vi "Read_binary_data.vi"() -> (1 "PWA Binary":i16[][](array[numeric]), 3 "PWA Frequency Hz":dbl format="%.2f", 5 "EOF?":bool, 6 "Block Header":string)   [LabVIEW 2022 SP3]
uses:
  Controls/Read I16 data cluster.ctl
  Globals/Meas_global.vi
  Globals/LDA_global.vi
panel:
  out "svnBaseRevision":u32
  out "string":string
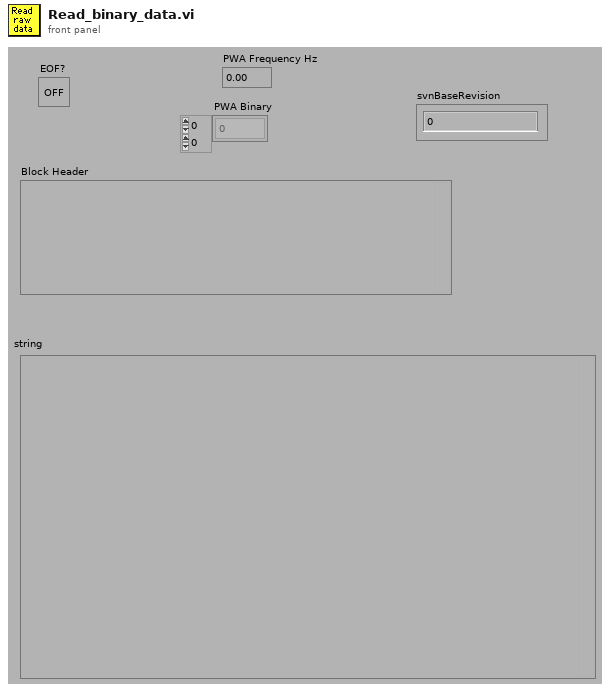
[diagram p1: front panel]
types:
  T1 = typedef "Analysis_info_cluster.ctl" = cluster{"Colour":u32, "Inst type":T2, "Inst name":string, "Symbol":string, "Code name":string, "Extra Info":string, "Inst Array":T3, "U":dbl, "u^2":dbl, "u^3":dbl, "u^4":dbl, "Skew_u":dbl, "Kurt_u":dbl, "Sd Error in Mean":dbl, "% u'/U":dbl, "X":dbl, "Y":dbl, "Z":dbl, "Timescale integral Estimate":dbl, "Sd Error in Variance":dbl, "Calib File":path, "Calib Constants":dbl[], "Output Position":bool, "Stats":enum16{"None", "Basic", "Full"}, "Av Sampling Rate":dbl, "Av No of Samples":dbl, "Total Meas Time (s)":dbl, "OrigChName":string, "Max value":dbl, "Min value":dbl, "Req Sample Rate Hz":dbl, "Sync Delay Time (s)":dbl, "Ch No":i16, "Device":string, "Use Latest Calib":bool, "Port":string, "Metadata Ch Names":string[], "Metadata Ch Values":string[], "Label":string, "chState":T4, "Point Drift":dbl, "inputConfig":string}
  T2 = typedef "Inst_type.ctl" = enum16{"Raw voltage", "Raw with zero offsetting", "Propeller anemometer", "Pressure Transducer", "Pitot-static tube", "Hot wire", "Cross wire 1", "Cross wire 2", "Generic Linear", "Generic Polynomial", "Generic BackPoly", "Fast FID", "Thermocouple", "Cold wire", "Pulsed Wire", "LDA Vel", "LDA Tran time", "LDA Arr time", "Microphone"}
  T3 = typedef "Instrument_Array.ctl" = enum16{"PWA", "LDA", "Analogue"}
  T4 = typedef "channelState.ctl" = enum32{"No Selection", "Solo", "Mute"}
  T5 = enum16{"read/write", "read-only", "write-only", "write-only (truncate)"}
  T6 = typedef "Read I16 data cluster.ctl" = cluster{"scale multiplier":dbl, "scale offset":dbl, "Length":i32, "Sampling rate (Hz)":dbl, "Sync Delay (s)":dbl}
  T7 = typedef "BSA_Type.ctl" = enum16{"57N11", "BSA F60"}
  T8 = typedef "PWA_Data.ctl" = enum16{"No PWA Data", "One Ch PWA"}
  T9 = typedef "Time_Trace_Cluster.ctl" = cluster{"Weighting":dbl[], "Voltage":dbl[], "Eng Values":dbl[]}
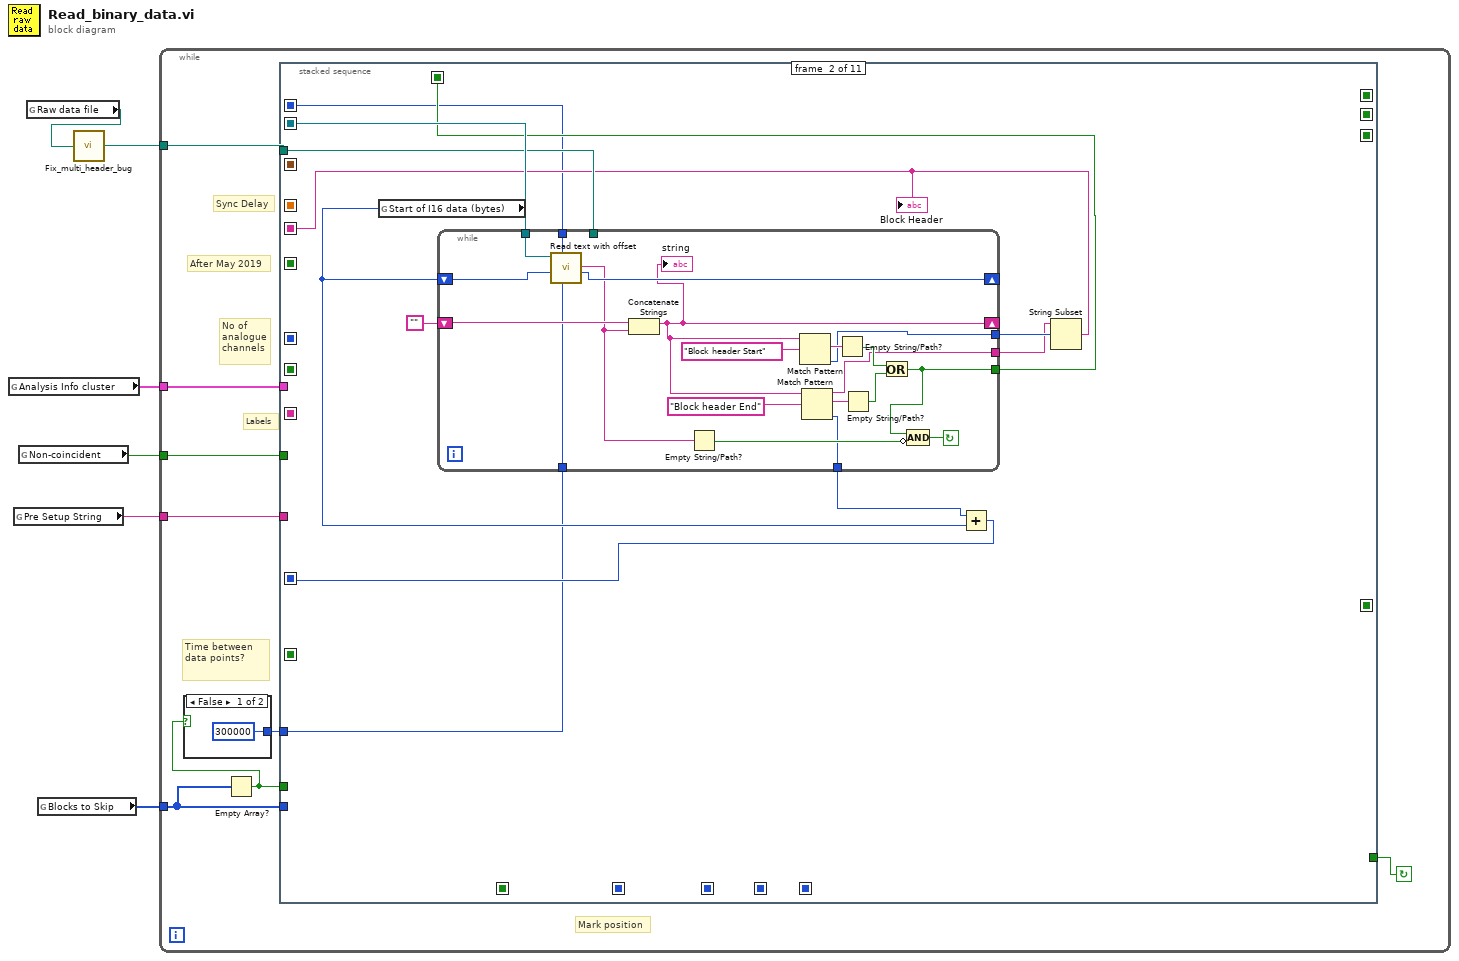
[diagram p0: block diagram]
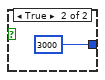
[diagram p2: hidden frame]
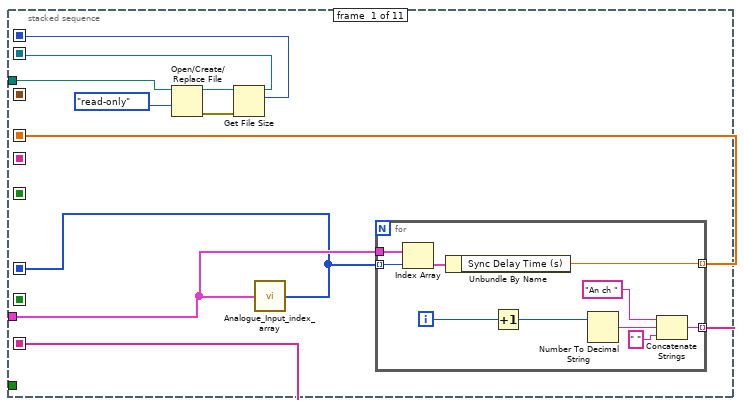
[diagram p3: hidden frame]
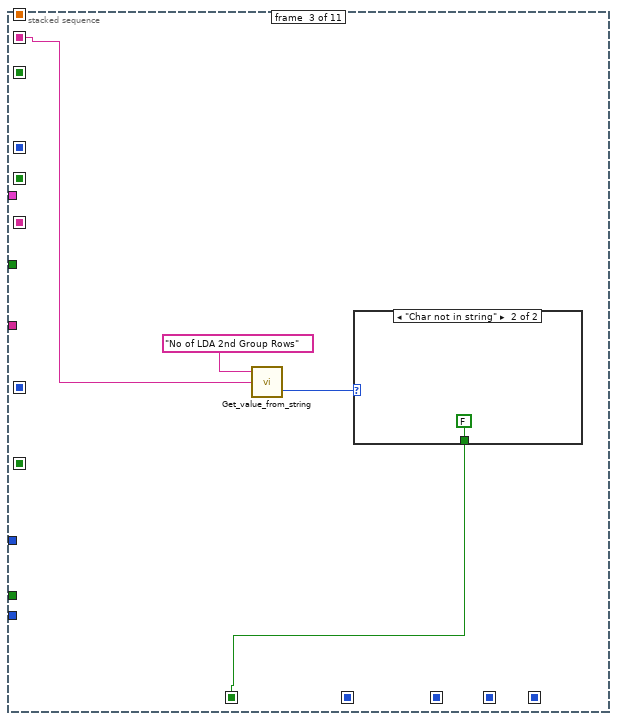
[diagram p4: hidden frame]
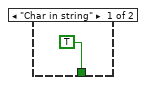
[diagram p5: hidden frame]
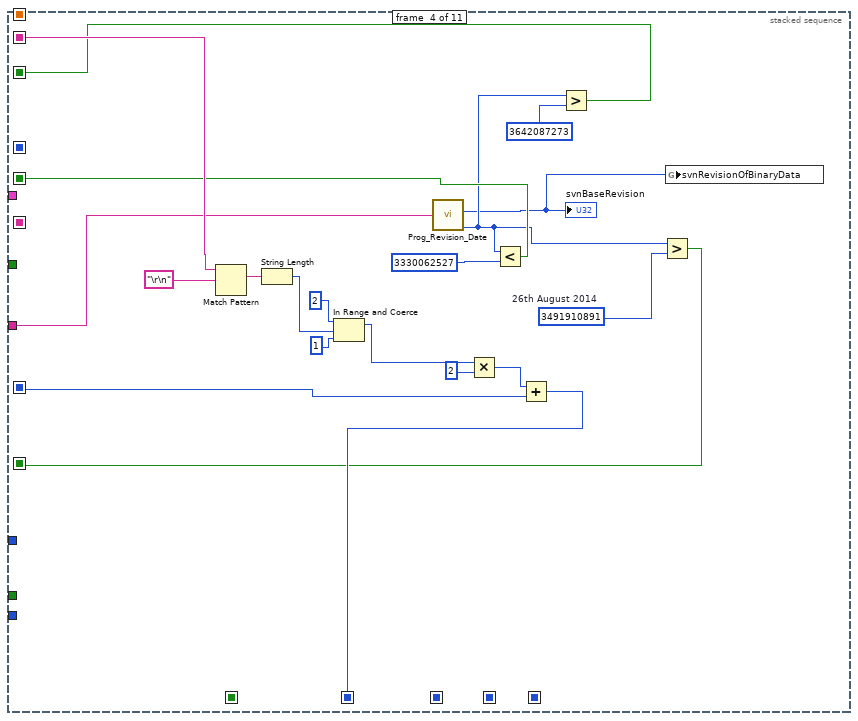
[diagram p6: hidden frame]
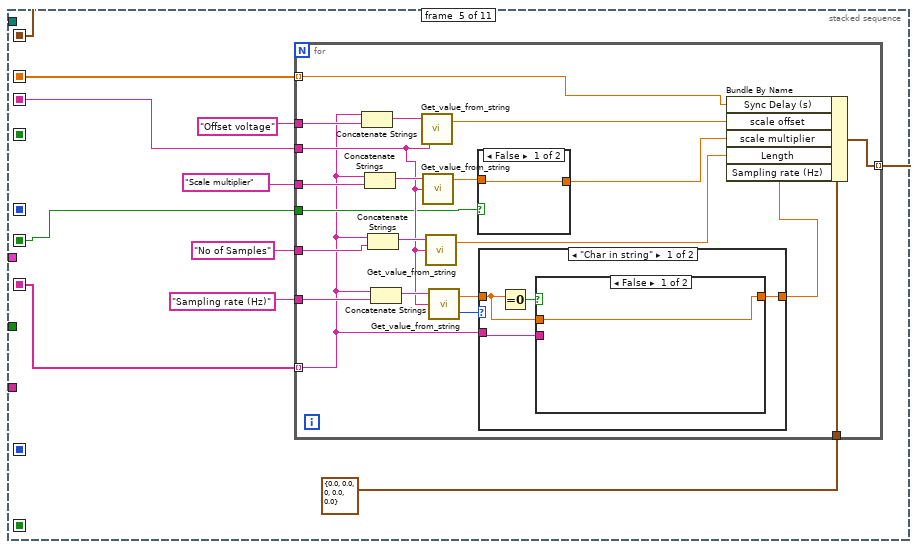
[diagram p7: hidden frame]
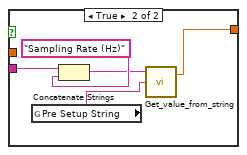
[diagram p8: hidden frame]
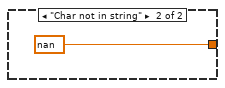
[diagram p9: hidden frame]
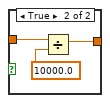
[diagram p10: hidden frame]
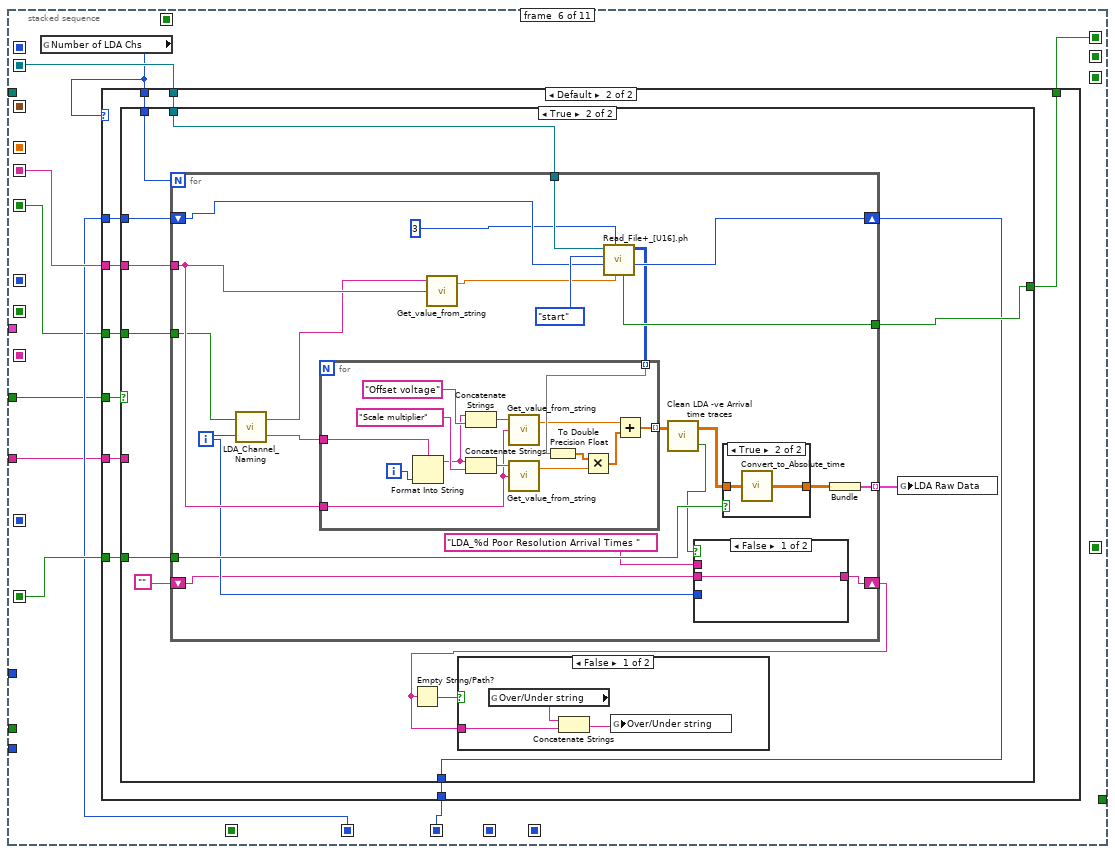
[diagram p11: hidden frame]
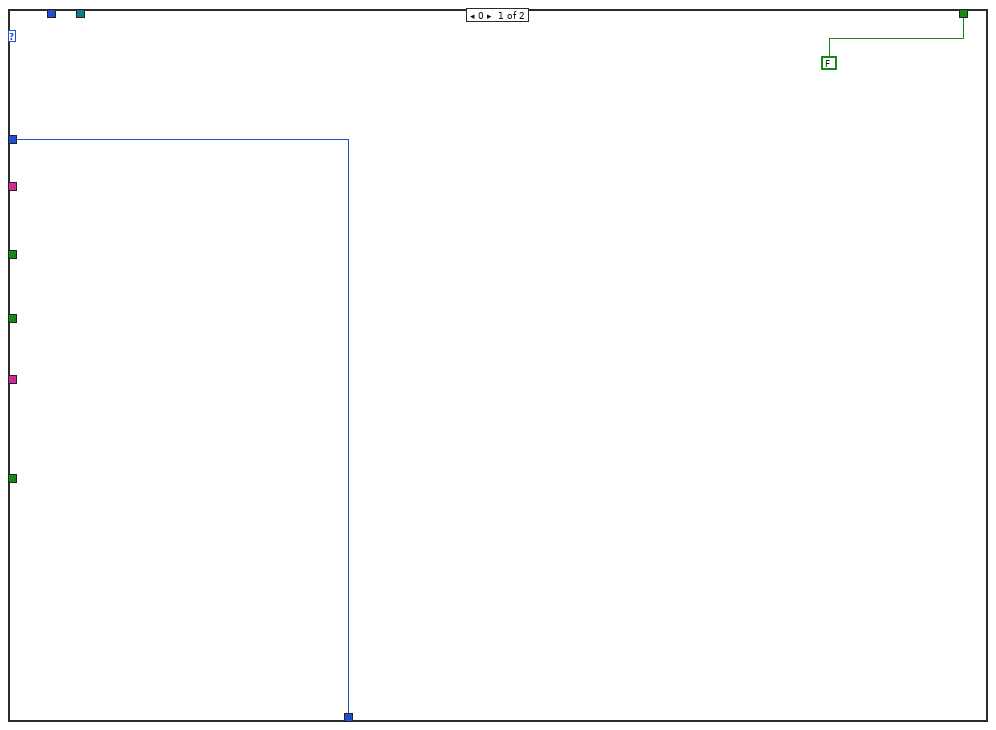
[diagram p12: hidden frame]
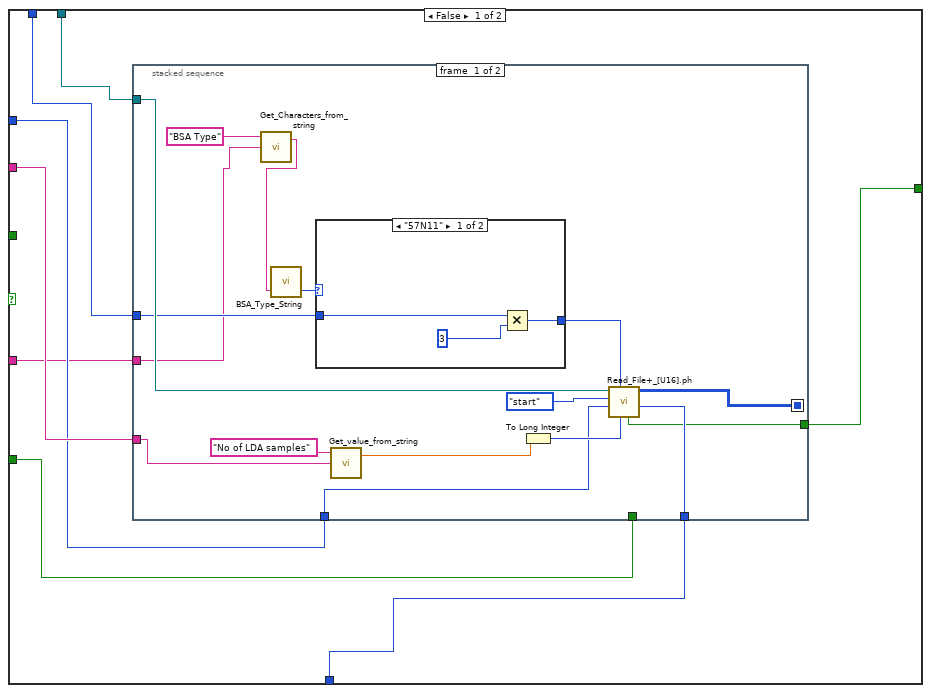
[diagram p13: hidden frame]
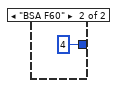
[diagram p14: hidden frame]
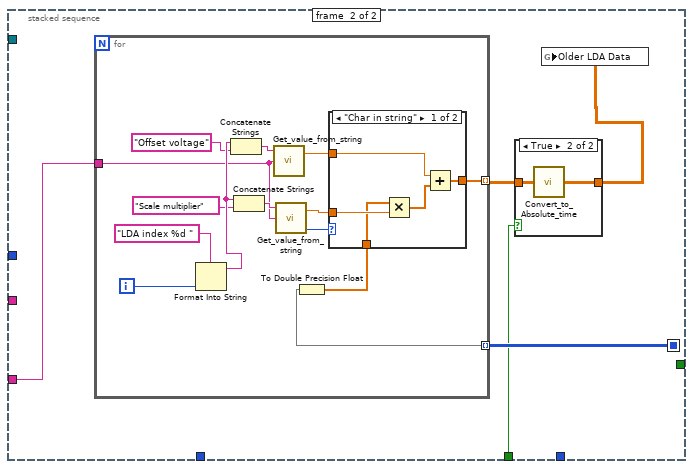
[diagram p15: hidden frame]
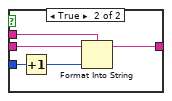
[diagram p19: hidden frame]
diagram:
  n1 = global read "Meas_global.vi" "Analysis Info cluster"() -> (w4:T1[])
  n2 = global read "Meas_global.vi" "Pre Setup String"() -> (w2:string)
  n3 = global read "LDA_global.vi" "Non-coincident"() -> (w3:bool)
  n4 = global read "Meas_global.vi" "Raw data file"() -> (w6:path)
  n5 = global read "Meas_global.vi" "Blocks to Skip"() -> (w1:i32[])
  n6 = call "Fix_multi_header_bug.vi"("Raw data File to Read"=w6) -> ("Raw data File to Read Out"=w5:path)
  n7 = while {
    tunnel: w5 -> [w14]
    tunnel: w4 -> [w12]
    tunnel: w3 -> [w11]
    tunnel: w2 -> [w10]
    tunnel: w1 -> [w9]
    stop <- w13 continue-if-true
    # "After May 2019"
    # "Sync Delay"
    # "Time between data points?"
    # "Mark position"
    # "Labels"
    # "No of\nanalogue\nchannels"
    n8 = Empty Array?(array=w9) -> (empty?=w8:bool)
    n9 = case shown="False" w8 {
      tunnel: [300000 3000] -> w7
      frame False {
      }
      frame True {
      }
    }
    n10 = stacked-sequence {
      seq-local: [w19 _ _ _ _ _ _ _ _ _ _] -> [_ w48 _ _ _ w148 w286 w325 _ w361 w416]
      seq-local: [_ w39 _ _ _ _ _ _ _ _ _] -> [_ _ w71 w88 w100 w149 w288 w320 w341 _ _]
      seq-local: [w21 _ _ _ _ _ _ _ _ _ _] -> [_ _ _ _ _ _ _ w319 _ _ _]
      seq-local: [w24 _ _ _ _ _ _ _ _ _ _] -> [_ _ _ _ w102 _ _ _ _ _ _]
      seq-local: [_ _ _ w92 _ _ _ _ _ _ _] -> [_ _ _ _ _ w147 _ _ _ _ _]
      seq-local: [_ _ _ _ _ w145 _ _ _ _ _] -> [_ _ _ _ _ _ w281 _ _ _ _]
      seq-local: [_ _ _ _ _ _ w287 _ _ _ _] -> [_ _ _ _ _ _ _ w323 _ _ _]
      seq-local: [_ w44 _ _ _ _ _ _ _ _ _] -> [_ _ _ _ _ _ _ _ _ _ w417]
      seq-local: [_ w43 _ _ _ _ _ _ _ _ _] -> [_ _ _ w93 _ _ _ _ _ _ _]
      seq-local: [_ _ _ _ _ _ _ _ w340 _ _] -> [_ _ _ _ _ _ _ _ _ w354 _]
      seq-local: [_ _ _ _ _ _ _ w322 _ _ _] -> [_ _ _ _ _ _ _ _ _ w358 _]
      seq-local: [_ _ w69 _ _ _ _ _ _ _ _] -> [_ _ _ _ _ _ _ _ _ _ _]
      seq-local: [_ _ _ w81 _ _ _ _ _ _ _] -> [_ _ _ _ _ w150 _ _ _ _ _]
      seq-local: [_ _ _ w80 _ _ _ _ _ _ _] -> [_ _ _ _ w99 _ _ _ _ _ _]
      seq-local: [_ _ _ _ w96 _ _ _ _ _ _] -> [_ _ _ _ _ _ _ w316 _ _ _]
      seq-local: [w23 _ _ _ _ _ _ _ _ _ _] -> [_ _ _ _ w95 _ _ _ _ _ _]
      seq-local: [_ _ _ w77 _ _ _ _ _ _ _] -> [_ _ _ _ _ w146 _ _ _ _ _]
      seq-local: [w17 _ _ _ _ _ _ _ _ _ _] -> [_ w38 _ _ _ _ _ _ _ w359 _]
      seq-local: [_ _ _ _ _ w141 _ _ _ _ _] -> [_ _ _ _ _ _ w279 _ _ _ _]
      seq-local: [_ _ _ _ _ _ w280 _ _ _ _] -> [_ _ _ _ _ _ _ w314 _ _ _]
      seq-local: [_ _ _ _ _ _ _ w315 _ _ _] -> [_ _ _ _ _ _ _ _ _ w356 _]
      tunnel: w14 -> [w25 w47 _ _ _ _ _ _ _ w360 w418]
      tunnel: [_ _ _ _ _ _ _ _ _ w353 _] -> w13
      tunnel: w12 -> [w22 _ _ _ _ _ _ _ _ _ _]
      tunnel: w11 -> [_ _ _ _ _ w144 _ _ _ _ _]
      tunnel: w10 -> [_ _ _ w76 _ w143 _ _ _ _ _]
      tunnel: w9 -> [_ _ _ _ _ _ _ _ w339 w352 _]
      tunnel: w8 -> [_ _ _ _ _ _ _ _ w338 w351 _]
      tunnel: w7 -> [_ w37 _ _ _ _ _ _ _ w350 _]
      frame #0 {
        n11 = Open/Create/Replace File(file path (use dialog)=w25, access (0:read/write)=T5."read-only" ("open mode (0)")) -> (refnum out=w20:refnum<file>, error out=w18:errorcluster)  [unwired: 1 in, 4 out]
        n12 = Get File Size(file=w20, error in=w18) -> (refnum out=w19:refnum<file>, size (in bytes)=w17:i64)  [unwired: 1 out]
        n13 = call "Analogue_Input_index_array.vi"("Analysis Info cluster"=w22) -> ("Array"=w21:i32[])
        n14 = for {
          tunnel: [w35] -> w24 mode=indexing
          tunnel: [w34] -> w23 mode=indexing
          tunnel: w22 -> [w29]
          tunnel: w21 -> [w28] mode=indexing
          i -> [w36]
          n15 = Index Array(array=w29, index=w28) -> (element=w27:T1)
          n16 = Unbundle By Name(w27) -> ("Sync Delay Time (s)"=w34:dbl)
          n17 = Increment(x=w36) -> (x+1=w31:i32)
          n18 = Number To Decimal String(number=w31) -> (decimal integer string=w33:string)  [unwired: 1 out]
          n19 = Concatenate Strings("An ch ", w33, " ") -> (w35:string)
        }
      }
      frame #1 {
        n20 = global read "Meas_global.vi" "Start of I16 data (bytes)"() -> (w45:i64)
        n21 = while {
          tunnel: [w55] -> w42
          tunnel: [w56] -> w44
          shift-left: "" -> [w59]
          shift-right: [w52] -> _
          tunnel: w47 -> [_]
          tunnel: w48 -> [w66]
          shift-left: w45 -> [w62]
          shift-right: [w65] -> _
          tunnel: [w54] -> w40
          tunnel: [w51] -> w41
          tunnel: w38 -> [w50]
          tunnel: w37 -> [w49]
          stop <- w63 continue-if-true
          n22 = call "Read text with offset.vi"("Count"=w49, "File Size"=w50, "Start of read offset (chars.: 0)"=w62, "Refnum In"=w66) -> ("Mark after Read"=w65:i64, "text"=w53:string)  [unwired: 3 in, 3 out]
          n23 = Concatenate Strings(w59, w53) -> (w52:string)
          "string" <- w52
          n24 = Empty String/Path?(string/path=w53) -> (empty?=w64:bool)
          n25 = Match Pattern(string=w52, regular expression="Block header Start") -> (match substring=w61:string, offset past match=w51:i32)  [unwired: 3 out]
          n26 = Match Pattern(string=w52, regular expression="Block header End") -> (before substring=w54:string, match substring=w67:string, offset past match=w55:i32)  [unwired: 2 out]
          n27 = Empty String/Path?(string/path=w61) -> (empty?=w58:bool)
          n28 = Empty String/Path?(string/path=w67) -> (empty?=w57:bool)
          n29 = Or(x=w58, y=w57) -> (x .or. y?=w56:bool)
          n30 = Compound Arithmetic op=AND(w56, invert w64) -> (w63:bool)
        }
        n31 = Add(x=w42, y=w45) -> (x+y=w43:i64)
        n32 = String Subset(string=w40, offset (0)=w41) -> (substring=w39:string)  [unwired: 1 out]
        "Block Header" <- w39
      }
      frame #2 {
        n33 = call "Get_value_from_string.vi"("Input string"=w71, "Variable name"="No of LDA 2nd Group Rows") -> ("Status"=w70:enum16{"Char in string", "Char not in string"})  [unwired: 1 in, 1 out]
        n34 = case shown="\"Char not in string\"" w70 {
          tunnel: [TRUE FALSE] -> w69
          frame "Char in string" {
          }
          frame "Char not in string" {
          }
        }
      }
      frame #3 {
        w82 = u32 3491910891  # 26th August 2014
        n35 = Match Pattern(string=w88, regular expression="\r\n") -> (match substring=w87:string)  [unwired: 4 out]
        n36 = String Length(string=w87) -> (length=w86:i32)
        n37 = In Range and Coerce(upper limit=2, x=w86, lower limit=1) -> (coerced(x)=w85:i32)  [unwired: 1 out]
        n38 = call "Prog_Revision_Date.vi"("Input string"=w76) -> ("Revision time (s)"=w79:u32, "svnBaseRevision"=w75:u32)  [unwired: 3 out]
        "svnBaseRevision" <- w75
        n39 = Multiply(x=w85, y=2) -> (x*y=w91:i32)
        n40 = Less?(x=w79, y=u32 3330062527 ("unsigned 32bit integer")) -> (x < y?=w80:bool)
        n41 = Add(x=w91, y=w93) -> (x+y=w92:i64)
        n42 = Greater?(x=w79, y=u32 3642087273 ("unsigned 32bit integer")) -> (0:w77:bool)
        n43 = Greater?(x=w79, y=w82) -> (0:w81:bool)
        n44 = global write "Meas_global.vi" "svnRevisionOfBinaryData"(w75) -> ()
      }
      frame #4 {
        n45 = for {
          tunnel: "Scale multiplier" -> [w125]
          tunnel: "Offset voltage" -> [w124]
          tunnel: w100 -> [w116]
          tunnel: w102 -> [w106] mode=indexing
          tunnel: T6 {"scale multiplier"=0.0, "scale offset"=0.0, "Length"=0, "Sampling rate (Hz)"=0.0, "Sync Delay (s)"=0.0} -> [w121]
          tunnel: "Sampling rate (Hz)" ("string") -> [w118]
          tunnel: "No of Samples" -> [w117]
          tunnel: w99 -> [w115]
          tunnel: [w108] -> w96 mode=indexing
          tunnel: w95 -> [w107] mode=indexing
          n46 = Concatenate Strings(w106, w124) -> (w123:string)
          n47 = Concatenate Strings(w106, w125) -> (w122:string)
          n48 = Concatenate Strings(w106, w117) -> (w120:string)
          n49 = Concatenate Strings(w106, w118) -> (w119:string)
          n50 = call "Get_value_from_string.vi"("Input string"=w116, "Variable name"=w123) -> ("Value"=w113:dbl)  [unwired: 1 in, 1 out]
          n51 = call "Get_value_from_string.vi"("Input string"=w116, "Variable name"=w122) -> ("Value"=w114:dbl)  [unwired: 1 in, 1 out]
          n52 = call "Get_value_from_string.vi"("Input string"=w116, "Variable name"=w120) -> ("Value"=w111:dbl)  [unwired: 1 in, 1 out]
          n53 = call "Get_value_from_string.vi"("Input string"=w116, "Variable name"=w119) -> ("Status"=w110:enum16{"Char in string", "Char not in string"}, "Value"=w109:dbl)  [unwired: 1 in]
          n54 = case shown="False" w115 {
            tunnel: w114 -> [w137 w140]
            tunnel: [w137 w138] -> w112
            frame False {
            }
            frame True {
              n55 = Divide(x=w140, y=10000.0) -> (x/y=w138:dbl)
            }
          }
          n56 = case shown="\"Char in string\"" w110 {
            tunnel: [w127 nan ("Value")] -> w105
            tunnel: w109 -> [w126 _]
            tunnel: w106 -> [w129 _]
            frame "Char in string" {
              n57 = Equal To 0?(x=w126) -> (x = 0?=w128:bool)
              n58 = case shown="False" w128 {
                tunnel: w129 -> [_ w135]
                tunnel: [w130 w131] -> w127
                tunnel: w126 -> [w130 _]
                frame False {
                }
                frame True {
                  n59 = global read "Meas_global.vi" "Pre Setup String"() -> (w133:string)
                  n60 = Concatenate Strings(w135, "Sampling Rate (Hz)" ("string")) -> (w132:string)
                  n61 = call "Get_value_from_string.vi"("Input string"=w133, "Variable name"=w132) -> ("Value"=w131:dbl)  [unwired: 1 in, 1 out]
                }
              }
            }
            frame "Char not in string" {
            }
          }
          n62 = Bundle By Name(cluster=w121, "Sync Delay (s)"=w107, "scale offset"=w113, "scale multiplier"=w112, "Length"=w111, "Sampling rate (Hz)"=w105) -> (w108:T6)
        }
      }
      frame #5 {
        n63 = global read "LDA_global.vi" "Number of LDA Chs"() -> (w142:i32)
        n64 = case shown="Default" w142 {
          tunnel: w150 -> [_ w162]
          tunnel: w149 -> [_ w161]
          tunnel: w148 -> [_ w160]
          tunnel: w147 -> [w152 w159]
          tunnel: w146 -> [_ w158]
          tunnel: [w152 w157] -> w145
          tunnel: w144 -> [_ w156]
          tunnel: w142 -> [_ w155]
          tunnel: w143 -> [_ w154]
          tunnel: [FALSE ("EOF?") w153] -> w141
          frame 0 {
          }
          frame Default {
            n65 = case shown="True" w156 {
              tunnel: w162 -> [w165 w230]
              tunnel: w161 -> [w167 w228]
              tunnel: w160 -> [w170 w227]
              tunnel: w159 -> [w166 w226]
              tunnel: w158 -> [_ w225]
              tunnel: [w169 w223] -> w157
              tunnel: [w168 w224] -> w153
              tunnel: w155 -> [w164 w222]
              tunnel: w154 -> [w163 _]
              frame False {
                n66 = stacked-sequence {
                  seq-local: [w178 _] -> [_ w194]
                  tunnel: w170 -> [w186 _]
                  tunnel: w166 -> [w180 _]
                  tunnel: w167 -> [w174 w195]
                  tunnel: [w179 _] -> w169
                  tunnel: w165 -> [_ w192]
                  tunnel: [w177 _] -> w168
                  tunnel: w164 -> [w175 _]
                  tunnel: w163 -> [w173 _]
                  frame #0 {
                    n67 = call "Get_Characters_from_string.vi"("Input string"=w173, "Variable name"="BSA Type" ("Label for characters")) -> ("Value"=w172:string)  [unwired: 1 in, 1 out]
                    n68 = call "BSA_Type_String.vi"("BSA String in"=w172) -> ("BSA Type Out"=w171:T7)  [unwired: 1 in, 1 out]
                    n69 = case shown="\"57N11\"" w171 {
                      tunnel: [w189 4] -> w181
                      tunnel: w175 -> [w187 _]
                      frame "57N11" {
                        n70 = Multiply(x=w187, y=3) -> (x*y=w189:i32)
                      }
                      frame "BSA F60" {
                      }
                    }
                    n71 = call "Get_value_from_string.vi"("Input string"=w174, "Variable name"="No of LDA samples") -> ("Value"=w184:dbl)  [unwired: 1 in, 1 out]
                    n72 = To Long Integer(number=w184) -> (32bit integer=w182:i32)
                    n73 = call "Read_File+_[U16].ph.vi"("2D number of columns/1D count"=w182, "2D number of rows"=w181, "pos offset (bytes:0)"=w180, "pos mode (rel. to current:2)"=enum16{"start", "end", "current"}."start", "refnum"=w186) -> ("mark after read (bytes)"=w179:i32, "2D data"=w178:u16[][], "EOF?"=w177:bool)  [unwired: 1 in, 3 out]
                  }
                  frame #1 {
                    n74 = for {
                      tunnel: w195 -> [w204]
                      tunnel: w194 -> [w202] mode=indexing
                      tunnel: [w200] -> w193 mode=indexing
                      i -> [w203]
                      n75 = Format Into String(format string="LDA index %d ", w203) -> (resulting string=w209:string)  [unwired: 2 in, 1 out]
                      n76 = Concatenate Strings(w209, "Offset voltage") -> (w206:string)
                      n77 = Concatenate Strings(w209, "Scale multiplier") -> (w205:string)
                      n78 = call "Get_value_from_string.vi"("Input string"=w204, "Variable name"=w206) -> ("Value"=w210:dbl)  [unwired: 1 in, 1 out]
                      n79 = call "Get_value_from_string.vi"("Input string"=w204, "Variable name"=w205) -> ("Status"=w199:enum16{"Char in string", "Char not in string"}, "Value"=w212:dbl)  [unwired: 1 in]
                      n80 = To Double Precision Float(number=w202) -> (double precision float=w201:dbl[])
                      n81 = case shown="\"Char in string\"" w199 {
                        tunnel: w212 -> [w217 _]
                        tunnel: w210 -> [w216 _]
                        tunnel: w201 -> [w214 w218]
                        tunnel: [w213 w218] -> w200
                        frame "Char in string" {
                          n82 = Multiply(x=w214, y=w217) -> (x*y=w215:dbl[])
                          n83 = Add(x=w216, y=w215) -> (x+y=w213:dbl[])
                        }
                        frame "Char not in string" {
                        }
                      }
                    }
                    n84 = case shown="True" w192 {
                      tunnel: w193 -> [w196 w198]
                      tunnel: [w196 w197] -> w191
                      frame False {
                      }
                      frame True {
                        n85 = call "Convert_to_Absolute_time.vi"("LDA Group in"=w198) -> ("LDA Group out"=w197:dbl[][])
                      }
                    }
                    n86 = global write "LDA_global.vi" "Older LDA Data"(w191) -> ()
                  }
                }
              }
              frame True {
                n87 = for {
                  N: w222 -> [_]
                  tunnel: w230 -> [w253]
                  tunnel: [w251] -> w229 mode=indexing
                  tunnel: w228 -> [w250]
                  tunnel: w227 -> [w249]
                  shift-right: [w247] -> w223
                  shift-left: w226 -> [w248]
                  tunnel: w225 -> [w244]
                  tunnel: [w242] -> w224
                  shift-right: [w234] -> w219
                  shift-left: "" -> [w235]
                  i -> [w237]
                  n88 = call "LDA_Channel_Naming.vi"("Numeric"=w237, "After May 2019"=w244) -> ("Channel Name"=w246:string, "No of Samples"=w245:string)
                  n89 = call "Get_value_from_string.vi"("Input string"=w250, "Variable name"=w245) -> ("Value"=w254:dbl)  [unwired: 1 in, 1 out]
                  n90 = call "Read_File+_[U16].ph.vi"("2D number of columns/1D count"=w254, "2D number of rows"=3, "pos offset (bytes:0)"=w248, "pos mode (rel. to current:2)"=enum16{"start", "end", "current"}."start", "refnum"=w249) -> ("mark after read (bytes)"=w247:i32, "2D data"=w241:u16[][], "EOF?"=w242:bool)  [unwired: 1 in, 3 out]
                  n91 = for {
                    tunnel: w250 -> [w273]
                    tunnel: w241 -> [w267] mode=indexing
                    tunnel: [w269] -> w240 mode=indexing
                    tunnel: w246 -> [w268]
                    i -> [w270]
                    n92 = Format Into String(format string=w268, w270) -> (resulting string=w274:string)  [unwired: 2 in, 1 out]
                    n93 = Concatenate Strings(w274, "Offset voltage") -> (w277:string)
                    n94 = Concatenate Strings(w274, "Scale multiplier") -> (w278:string)
                    n95 = call "Get_value_from_string.vi"("Input string"=w273, "Variable name"=w277) -> ("Value"=w265:dbl)  [unwired: 1 in, 1 out]
                    n96 = call "Get_value_from_string.vi"("Input string"=w273, "Variable name"=w278) -> ("Value"=w266:dbl)  [unwired: 1 in, 1 out]
                    n97 = To Double Precision Float(number=w267) -> (double precision float=w272:dbl[])
                    n98 = Multiply(x=w272, y=w266) -> (x*y=w271:dbl[])
                    n99 = Add(x=w265, y=w271) -> (x+y=w269:dbl[])
                  }
                  n100 = call "Clean LDA -ve Arrival time traces.vi"("LDA Data In"=w240) -> ("Negative Arrival Time"=w238:bool, "LDA Data Out"=w239:dbl[][])  [unwired: 1 in]
                  n101 = case shown="False" w238 {
                    tunnel: w237 -> [_ w261]
                    tunnel: "LDA_%d Poor Resolution Arrival Times " ("format string") -> [_ w259]
                    tunnel: w235 -> [w256 w258]
                    tunnel: [w256 w257] -> w234
                    frame False {
                    }
                    frame True {
                      n102 = Increment(x=w261) -> (x+1=w260:i32)
                      n103 = Format Into String(format string=w259, initial string=w258, w260) -> (resulting string=w257:string)  [unwired: 1 in, 1 out]
                    }
                  }
                  n104 = case shown="True" w253 {
                    tunnel: w239 -> [w262 w264]
                    tunnel: [w262 w263] -> w252
                    frame False {
                    }
                    frame True {
                      n105 = call "Convert_to_Absolute_time.vi"("LDA Group in"=w264) -> ("LDA Group out"=w263:dbl[][])
                    }
                  }
                  n106 = Bundle("LDA Group out"=w252) -> (w251:cluster{"LDA Group out":dbl[][]})  [unwired: 1 in]
                }
                n107 = Empty String/Path?(string/path=w219) -> (empty?=w220:bool)
                n108 = case shown="False" w220 {
                  tunnel: w219 -> [w231 _]
                  frame False {
                    n109 = global read "Meas_global.vi" "Over/Under string"() -> (w233:string)
                    n110 = Concatenate Strings(w233, w231) -> (w232:string)
                    n111 = global write "Meas_global.vi" "Over/Under string"(w232) -> ()
                  }
                  frame True {
                  }
                }
                n112 = global write "LDA_global.vi" "LDA Raw Data"(w229) -> ()
              }
            }
          }
        }
      }
      frame #6 {
        n113 = global read "Meas_global.vi" "PWA Data"() -> (w284:T8)
        n114 = case shown="\"No PWA Data\"" w284 {
          tunnel: [0 1] -> w283
          frame "No PWA Data" {
          }
          frame "One Ch PWA" {
          }
        }
        n115 = Not Equal To 0?(x=w283) -> (x != 0?=w285:bool)
        n116 = case shown="True" w285 {
          tunnel: w288 -> [_ w295]
          tunnel: w281 -> [w293 w303]
          tunnel: [w293 w305] -> w287
          tunnel: w286 -> [_ w308]
          tunnel: w283 -> [_ w307]
          tunnel: [i16[][] [] ("2D array") w304] -> w282
          tunnel: [w291 w294] -> w280
          tunnel: w279 -> [w291 _]
          frame False {
          }
          frame True {
            w299 = FALSE  # Show Dialog?
            n117 = call "Get_Characters_from_string.vi"("Input string"=w295, "Variable name"="No of PWA samples") -> ("Value"=w302:string)  [unwired: 1 in, 1 out]
            n118 = Decimal String To Number(string=w302) -> (number=w301:i32)  [unwired: 3 out]
            n119 = call <vilib>:"Read File+ [I16].vi"("2D number of columns/1D count"=w301, "2D number of rows"=w307, "pos offset (bytes:0)"=w303, "pos mode (rel. to current:2)"=enum16{"start", "end", "current"}."start", "refnum"=w308) -> ("mark after read (bytes)"=w305:i32, "2D data"=w304:i16[][], "EOF?"=w294:bool)  [unwired: 1 in, 3 out]
            n120 = call "Get_value_from_string.vi"("Show Dialog?"=w299, "Input string"=w295, "Variable name"="ADC Frequency Hz") -> ("Status"=w296:enum16{"Char in string", "Char not in string"}, "Value"=w298:dbl)
            n121 = case shown="\"Char not in string\"" w296 {
              tunnel: w298 -> [w310 _]
              tunnel: [w310 w311] -> w297
              tunnel: w295 -> [_ w312]
              frame "Char in string" {
              }
              frame "Char not in string" {
                n122 = call "Get_value_from_string.vi"("Input string"=w312, "Variable name"="Actual sampling rate") -> ("Value"=w311:dbl)  [unwired: 1 in, 1 out]
              }
            }
            "PWA Frequency Hz" <- w297
          }
        }
        "PWA Binary" <- w282
      }
      frame #7 {
        n123 = global read "Meas_global.vi" "Time Trace"() -> (w318:T9[])
        n124 = Array Size(array=w319) -> (size(s)=w321:i32)
        n125 = Not Equal To 0?(x=w321) -> (x != 0?=w324:bool)
        n126 = case shown="True" w324 {
          tunnel: w320 -> [_ w330]
          tunnel: w323 -> [w328 w335]
          tunnel: [w328 w336] -> w322
          tunnel: w325 -> [_ w337]
          tunnel: w319 -> [_ w334]
          tunnel: w318 -> [w327 w333]
          tunnel: [w327 w332] -> w317
          tunnel: w316 -> [_ w331]
          tunnel: [w326 w329] -> w315
          tunnel: w314 -> [w326 _]
          frame False {
          }
          frame True {
            n127 = call "Read I16 analogue Data.vi"("Block Header"=w330, "Channel info"=w331, "Time Trace In"=w333, "Analogue Index"=w334, "pos offset (bytes:0)"=w335, "refnum"=w337) -> ("Time Trace out"=w332:T9[], "EOF?"=w329:bool, "mark after read (bytes)"=w336:i32)  [unwired: 3 in]
          }
        }
        n128 = global write "Meas_global.vi" "Time Trace"(w317) -> ()
      }
      frame #8 {
        n129 = case shown="False" w338 {
          tunnel: w341 -> [w347 _]
          tunnel: [w343 FALSE] -> w340
          tunnel: w339 -> [w342 _]
          frame False {
            n130 = call "Get_value_from_string.vi"("Input string"=w347, "Variable name"="Block No") -> ("Value"=w346:dbl)  [unwired: 1 in, 1 out]
            n131 = To Long Integer(number=w346) -> (32bit integer=w345:i32)
            n132 = Search 1D Array(1D array=w342, element=w345) -> (index of element=w344:i32)  [unwired: 1 out]
            n133 = Greater Or Equal To 0?(x=w344) -> (x >= 0?=w343:bool)
          }
          frame True {
          }
        }
      }
      frame #9 {
        n134 = case shown="False" w356 {
          selector: w356 -> [_ w413]
          tunnel: w361 -> [w370 _]
          tunnel: w360 -> [w369 _]
          tunnel: w359 -> [w368 _]
          tunnel: w358 -> [w367 w414]
          tunnel: w352 -> [w366 _]
          tunnel: [w365 w414] -> w357
          tunnel: [w364 w413] -> w355
          tunnel: w351 -> [w363 _]
          tunnel: w350 -> [w362 _]
          frame False {
            n135 = while {
              tunnel: w370 -> [w391]
              tunnel: w369 -> [w390]
              tunnel: w368 -> [w386]
              tunnel: w366 -> [w380]
              shift-right: [w379] -> _
              shift-left: w367 -> [w378]
              tunnel: [w378] -> w365
              tunnel: [w376] -> w364
              tunnel: w363 -> [w372]
              tunnel: w362 -> [w371]
              stop <- w373 continue-if-true
              n136 = while {
                tunnel: [w402] -> _
                shift-left: "" -> [w405]
                shift-right: [w399] -> _
                tunnel: w390 -> [_]
                tunnel: w391 -> [w410]
                shift-left: w378 -> [w394]
                shift-right: [w393] -> _
                tunnel: [w401] -> w387
                tunnel: [w398] -> w388
                tunnel: w386 -> [w397]
                tunnel: [w396] -> w377
                tunnel: [w395] -> w374
                tunnel: w372 -> [_]
                tunnel: w371 -> [w392]
                stop <- w408 continue-if-true
                n137 = call "Read text with offset.vi"("Count"=w392, "File Size"=w397, "Start of read offset (chars.: 0)"=w394, "Refnum In"=w410) -> ("Mark after Read"=w393:i64, "text"=w400:string, "EOF?"=w395:bool)  [unwired: 3 in, 2 out]
                n138 = Concatenate Strings(w405, w400) -> (w399:string)
                n139 = Empty String/Path?(string/path=w400) -> (empty?=w409:bool)
                n140 = Match Pattern(string=w399, regular expression="Block header Start") -> (match substring=w407:string, offset past match=w398:i32)  [unwired: 3 out]
                n141 = Match Pattern(string=w399, regular expression="Block header End") -> (before substring=w401:string, match substring=w411:string, offset past match=w396:i32)  [unwired: 2 out]
                n142 = Empty String/Path?(string/path=w407) -> (empty?=w404:bool)
                n143 = Empty String/Path?(string/path=w411) -> (empty?=w403:bool)
                n144 = Or(x=w404, y=w403) -> (x .or. y?=w402:bool)
                n145 = Compound Arithmetic op=AND(w402, invert w409, invert w395) -> (w408:bool)
              }
              n146 = String Subset(string=w387, offset (0)=w388) -> (substring=w381:string)  [unwired: 1 out]
              n147 = call "Get_value_from_string.vi"("Input string"=w381, "Variable name"="Block No") -> ("Value"=w384:dbl)  [unwired: 1 in, 1 out]
              n148 = To Long Integer(number=w384) -> (32bit integer=w383:i32)
              n149 = Search 1D Array(1D array=w380, element=w383) -> (index of element=w382:i32)  [unwired: 1 out]
              n150 = Greater Or Equal To 0?(x=w382) -> (x >= 0?=w375:bool)
              n151 = Compound Arithmetic op=AND(invert w374, w375) -> (w373:bool)
              n152 = Less Than 0?(x=w377) -> (x < 0?=w376:bool)
              n153 = Add(x=w378, y=w377) -> (x+y=w379:i64)
            }
          }
          frame True {
          }
        }
        "EOF?" <- w355
        n154 = global write "Meas_global.vi" "Start of I16 data (bytes)"(w357) -> ()
        n155 = Compound Arithmetic op=AND(w354, invert w355) -> (w353:bool)
      }
      frame #10 {
        n156 = Close File(refnum=w416) -> (error out=w415:errorcluster)  [unwired: 1 in, 1 out]
        n157 = case shown="True" w417 {
          tunnel: w418 -> [w420 _]
          tunnel: w415 -> [w419 _]
          frame False {
            n158 = call "Add_filename_to_err_message.vi"("error in (no error)"=w419, "Path"=w420) -> ("error out"=w421:errorcluster)
            n159 = call "EnFlo_Error_Handler.vi"("error in (no error)"=w421) -> ()  [unwired: 2 in, 3 out]
          }
          frame True {
            w425 = FALSE  # Dialog Box
            n160 = Bundle By Name(cluster=errorcluster {"status"=FALSE, "code"=0, "source"=""} ("error in (no error)"), "status"=TRUE ("Bundle Element"), "source"="The block header was not found in the file" ("Bundle Element")) -> (w426:errorcluster)
            n161 = call "EnFlo_Error_Handler.vi"("error in (no error)"=w426, "Error Type"="Raw Data File Error", "Dialog Box (F)"=w425) -> ()  [unwired: 3 out]
          }
        }
      }
    }
  }
